vi "Integrated File.vi"() -> ()   [LabVIEW 2021]
uses:
  <vilib>/MakerHub/LINX/Public/Sensors/Accelerometer/MPU60X0/DeviceAddresses.ctl
  <vilib>/MakerHub/LINX/Public/Sensors/Accelerometer/MPU60X0/Clock Source.ctl
  <vilib>/MakerHub/LINX/Public/Utilities/Open Serial.vi
  <vilib>/MakerHub/LINX/Public/Sensors/Motion/Servo/Servo Open One Channel.vi
  <vilib>/MakerHub/LINX/Public/Sensors/Motion/Servo/Servo Close One Channel.vi
  <vilib>/MakerHub/LINX/LMH-LINX.lvlib
  <vilib>/MakerHub/LINX/Public/Sensors/Accelerometer/MPU60X0/MPU60X0.lvlib
  <vilib>/MakerHub/LINX/Public/Sensors/Motion/Servo/Servo.lvlib
panel:
  in  "Ki X":dbl
  in  "Kd X":dbl
  in  "Kp X":dbl=1.0
  in  "Controller Type X":string(combo)="P"
  out "Acc Angle Y":dbl[](graph)=[nan]
  out "Acc Angle X":dbl[](graph)=[131.31801279400403]
  in  "Ki Y":dbl
  in  "Kd Y":dbl
  in  "Kp Y":dbl=1.0
  in  "Controller Type Y":string(combo)="P"
  out "Weighted Angle Y":dbl[](graph)=[nan]
  out "Weighted Angle X":dbl[](graph)=[131.31801279400403]
  in  "Alpha Y":dbl
  in  "Alpha X":dbl
  in  "Acc Offset Y":dbl[](array[numeric])=[90.0]
  in  "Acc Offset X":dbl[](array[numeric])=[30.0]
  in  "Reset":bool
  out "Gyro Angle X":dbl(graph)=10.372999999999987
  out "Gyro Angle Y":dbl(graph)=2.7879999999999896
  in  "Stop Button":bool
  out "Milliseconds to wait out":u32=1
  in  "Milliseconds to wait in":u32=1
  in  "Gyro Offset X":i16
  in  "Gyro Offset Y":i16
  in  "Serial Port":refnum<visa-resource-name>="COM8"
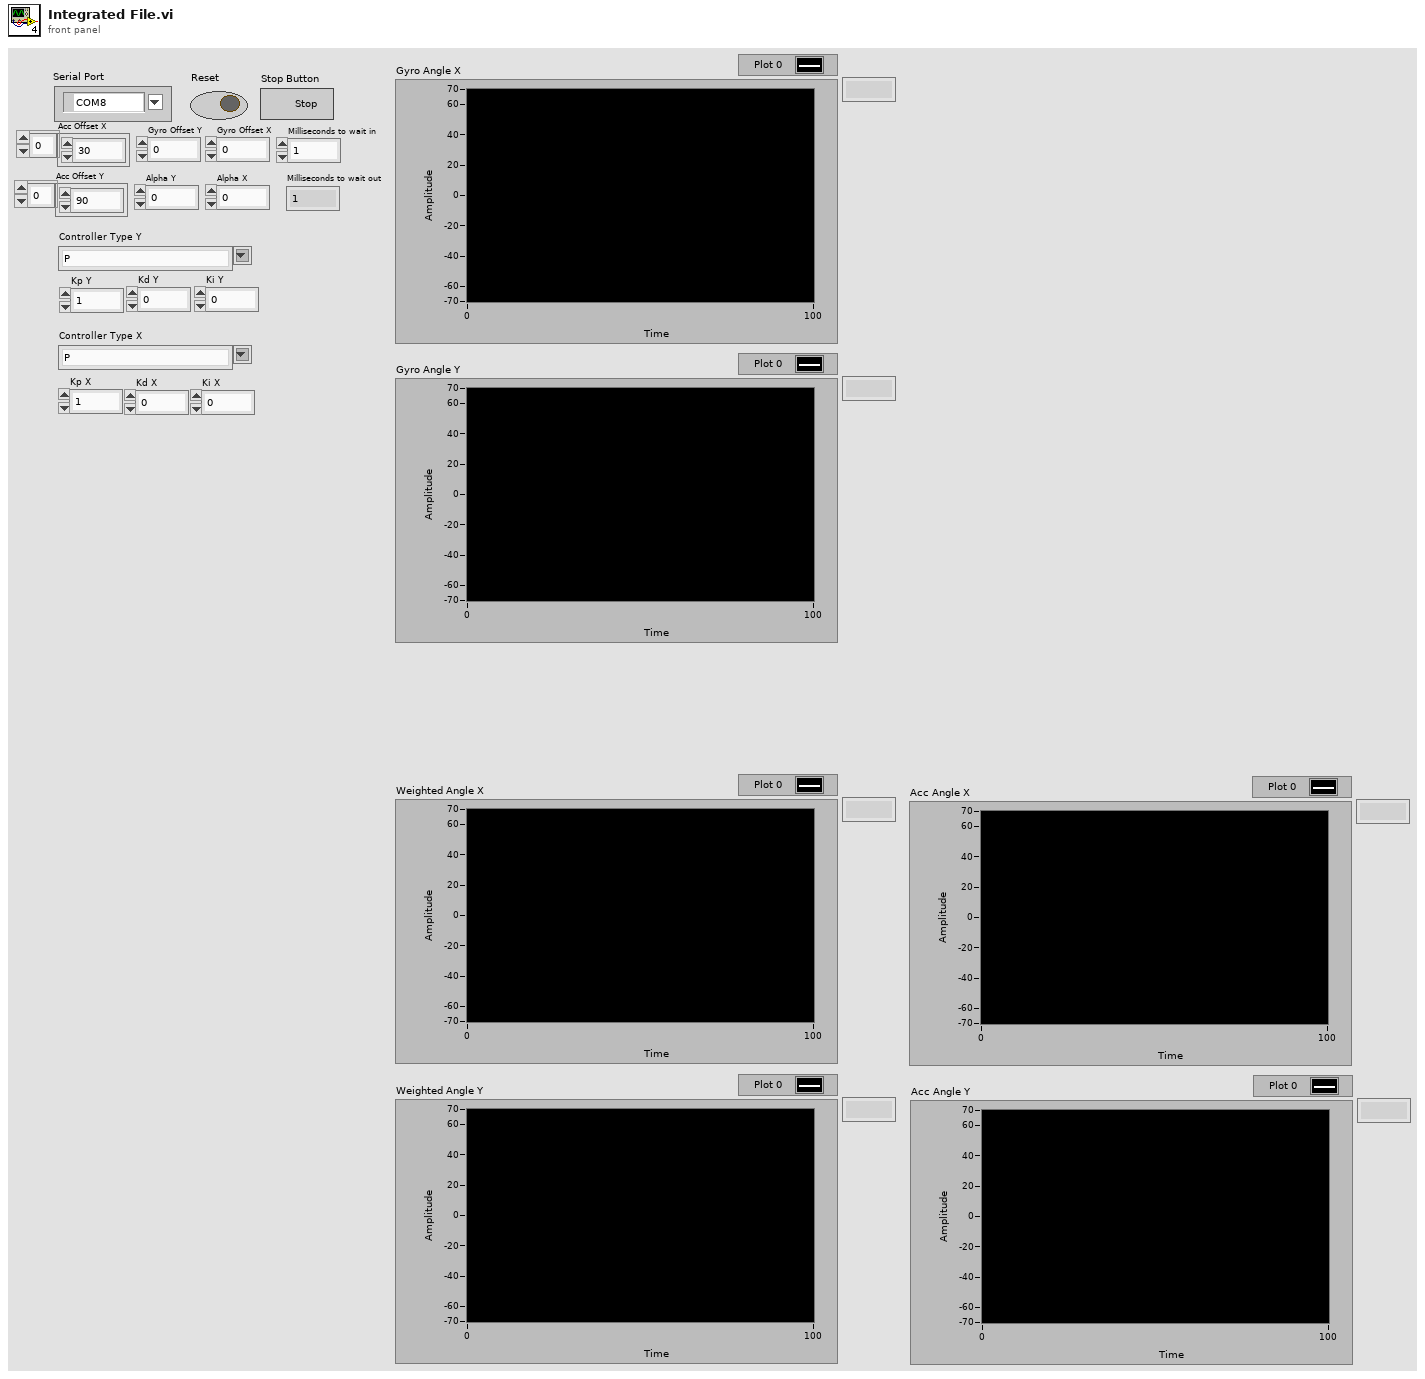
[diagram p1: front panel]
types:
  T1 = typedef "LMH-LINX.lvlib/MPU60X0.lvlib/Clock Source.ctl" = enum8{"Internal 8MHz Osc", "PLL with X Gyro Ref", "PLL with Y Gyro Ref", "PLL with Z Gyro Ref", "PLL with ext 32.768 KHz Ref", "PLL with ext 19.2 MHz Ref", "Reserved", "Hold in reset"}
  T2 = typedef "LMH-LINX.lvlib/MPU60X0.lvlib/DeviceAddresses.ctl" = enum16{"0x68", "0x69"}
  T3 = typedef "LMH-LINX.lvlib/LINX Ref.ctl" = cluster{"IO":T4, "Interface":T5, "LINX Device Config":T6}
  T4 = typedef "LMH-LINX.lvlib/Platform.ctl" = enum16{"Remote", "Local"}
  T5 = typedef "LMH-LINX.lvlib/Interface.ctl" = enum16{"Serial", "TCP"}
  T6 = typedef "LMH-LINX.lvlib/Device.lvlib/LINX Device Config.ctl" = cluster{"Interface":T5, "COM Port":refnum<visa-resource-name>, "TCP Configuration":T7, "Device Family":u8, "Device ID":u8, "Device Name":string, "TCP Ref":refnum<k5>, "Channels":T8}
  T7 = typedef "LMH-LINX.lvlib/Device.lvlib/TCP Config.ctl" = cluster{"IP Address":string, "Port":u16}
  T8 = typedef "LMH-LINX.lvlib/Channels.ctl" = cluster{"DI":u8[], "DO":u8[], "AI":u8[], "AO":u8[], "PWM":u8[], "QE":u8[], "UART":u8[], "I2C 2":u8[], "SPI":u8[], "CAN":u8[], "Servo":u8[], "AI Ref (V)":dbl, "AI Resolution (Bits)":u8, "AO Ref (V)":dbl, "AO Resolution (Bits)":u8}
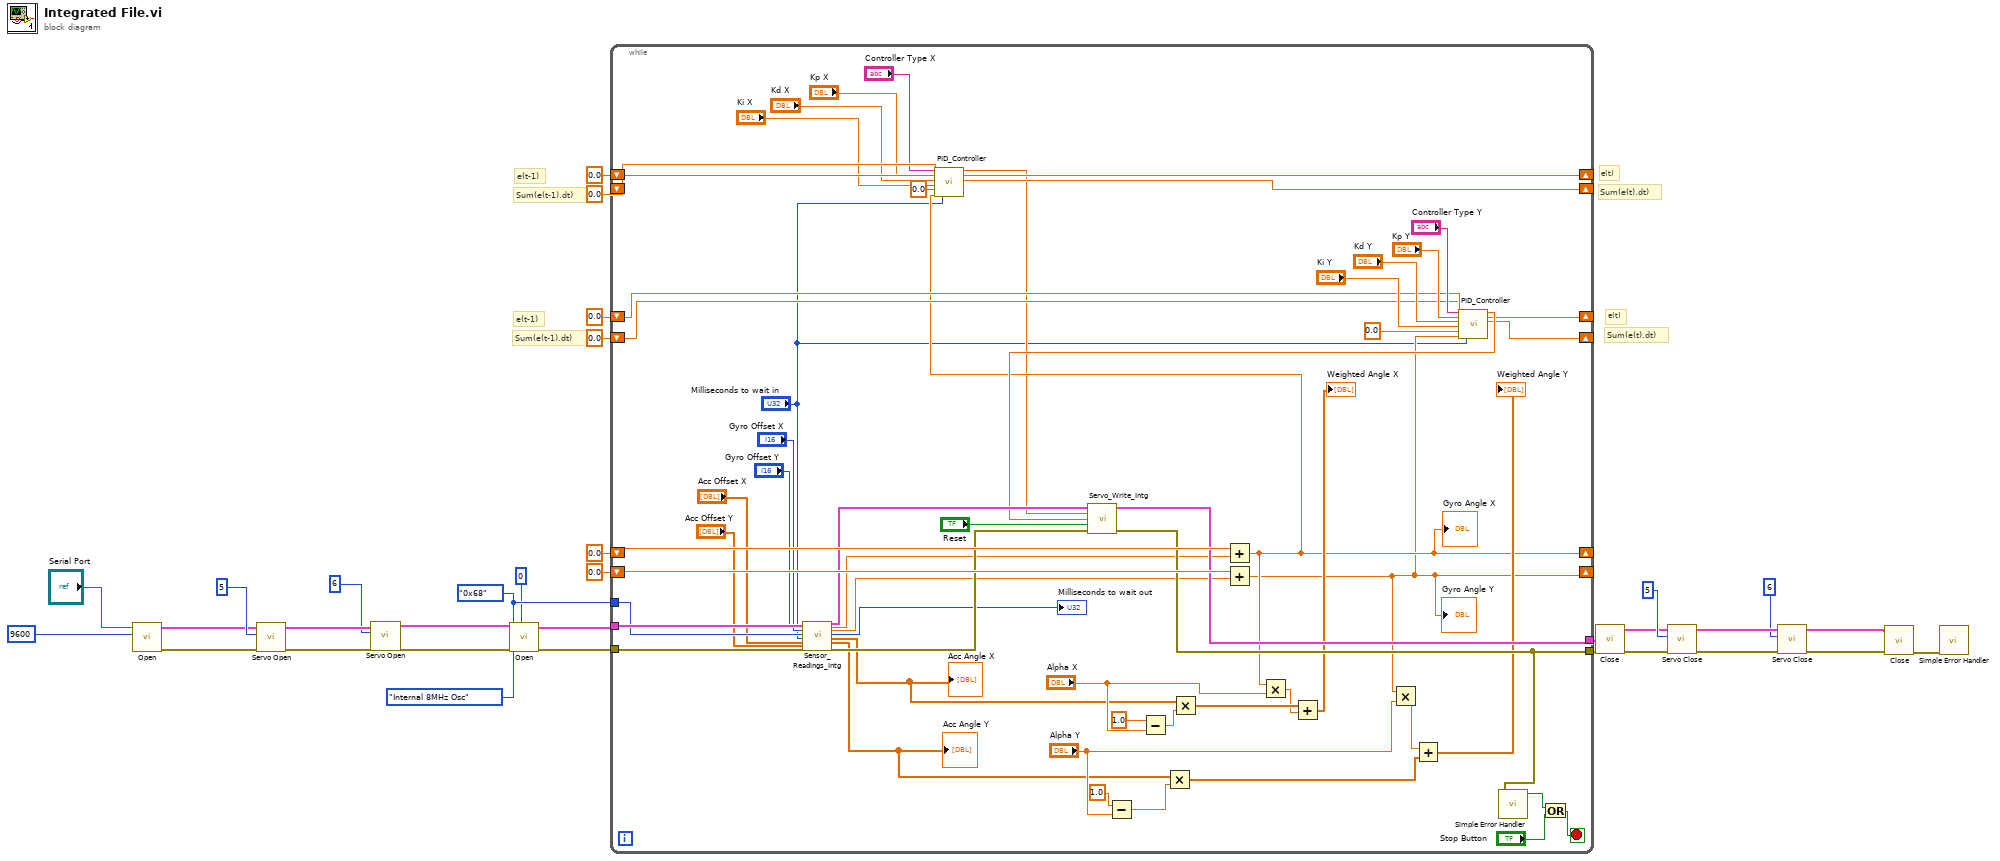
[diagram p0: block diagram]
diagram:
  w27 = DeviceAddresses."0x68" ("I2C Slave Address")
  # "Sum(e(t).dt)"
  # "e(t)"
  # "Sum(e(t-1).dt)"
  # "e(t-1)"
  # "Sum(e(t-1).dt)"
  # "e(t-1)"
  # "Sum(e(t).dt)"
  # "e(t)"
  n1 = call-poly <vilib>:"Open.vi"("Baud Rate Override"=u32 9600, "Serial Port"="Serial Port") -> ("Error Out"=w15:errorcluster, "LINX Resource"=w16:T3)  [unwired: 7 in, 1 out]
  n2 = call-poly <vilib>:"Servo Open.vi"("Error In"=w15, "Servo Channel"=u8 5, "LINX Resource"=w16) -> ("Error Out"=w19:errorcluster, "LINX Resource"=w20:T3)  [unwired: 7 in]
  n3 = call-poly <vilib>:"Servo Open.vi"("Error In"=w19, "Servo Channel"=u8 6, "LINX Resource"=w20) -> ("Error Out"=w13:errorcluster, "LINX Resource"=w14:T3)  [unwired: 7 in]
  n4 = call <vilib>:"Open.vi"("I2C Channel"=u8 0, "Error In"=w13, "Clock Source"=Clock_Source."Internal 8MHz Osc", "I2C Slave Address"=w27, "LINX Resource"=w14) -> ("Error Out"=w28:errorcluster, "LINX Resource"=w29:T3)  [unwired: 5 in]
  n5 = while {
    tunnel: w29 -> [w75]
    tunnel: w28 -> [w74]
    tunnel: w27 -> [w73]
    tunnel: [w84] -> w24
    tunnel: [w83] -> w23
    shift-right: [w36] -> _
    shift-left: 0.0 -> [w86]
    shift-right: [w34] -> _
    shift-left: 0.0 -> [w85]
    shift-right: [w42] -> _
    shift-left: 0.0 ("e(t)") -> [w45]
    shift-right: [w43] -> _
    shift-left: 0.0 ("e(t-1).dt+e(t).dt") -> [w44]
    shift-right: [w49] -> _
    shift-left: 0.0 ("e(t)") -> [w47]
    shift-right: [w48] -> _
    shift-left: 0.0 ("e(t-1).dt+e(t).dt") -> [w46]
    stop <- w87 stop-if-true
    n6 = call "Sensor_Readings_Intg.vi"("LINX Resource in"=w75, "Gyro Offset Y"="Gyro Offset Y", "Gyro Offset X"="Gyro Offset X", "I2C Slave Address"=w73, "Milliseconds to wait in"="Milliseconds to wait in", "Acc Offset X"="Acc Offset X", "Acc Offset Y"="Acc Offset Y", "error in (no error)"=w74) -> ("LINX Resource out"=w68:T3, "Gyro Angle X"=w66:dbl, "Gyro Angle Y"=w65:dbl, "Milliseconds to wait out"=→"Milliseconds to wait out":u32, "Acc Angle X"=w54:dbl[], "Acc Angle Y"=w53:dbl[], "error out"=w67:errorcluster)  [unwired: 13 in]
    "Acc Angle X" <- w54
    "Acc Angle Y" <- w53
    n7 = Subtract(x=1.0, y="Alpha Y") -> (x-y=w77:dbl)
    n8 = Subtract(x=1.0, y="Alpha X") -> (x-y=w81:dbl)
    n9 = Multiply(x=w53, y=w77) -> (x*y=w76:dbl[])
    n10 = Multiply(x=w54, y=w81) -> (x*y=w80:dbl[])
    n11 = Add(x=w86, y=w66) -> (x+y=w36:dbl)
    "Gyro Angle X" <- w36
    n12 = call "PID_Controller.vi"("Controller Type"="Controller Type X", "Kp"="Kp X", "Kd"="Kd X", "Ki"="Ki X", "Setpoint"=0.0, "Feedback Signal"=w36, "e(t-1).dt"=w44, "t"="Milliseconds to wait in", "e(t-1)"=w45) -> ("Control Signal"=w35:dbl, "e(t)"=w42:dbl, "e(t-1).dt+e(t).dt"=w43:dbl)  [unwired: 8 in]
    n13 = Add(x=w85, y=w65) -> (x+y=w34:dbl)
    "Gyro Angle Y" <- w34
    n14 = Multiply(x=w36, y="Alpha X") -> (x*y=w79:dbl)
    n15 = Add(x=w80, y=w79) -> (x+y=→"Weighted Angle X":dbl[])
    n16 = Multiply(x=w34, y="Alpha Y") -> (x*y=w78:dbl)
    n17 = Add(x=w78, y=w76) -> (x+y=→"Weighted Angle Y":dbl[])
    n18 = call "PID_Controller.vi"("Controller Type"="Controller Type Y", "Kp"="Kp Y", "Kd"="Kd Y", "Ki"="Ki Y", "Setpoint"=0.0, "Feedback Signal"=w34, "e(t-1).dt"=w46, "t"="Milliseconds to wait in", "e(t-1)"=w47) -> ("Control Signal"=w56:dbl, "e(t)"=w49:dbl, "e(t-1).dt+e(t).dt"=w48:dbl)  [unwired: 8 in]
    n19 = call "Servo_Write_Intg.vi"("LINX Resource in"=w68, "Servo X"=w35, "Servo Y"=w56, "Reset"="Reset", "error in (no error)"=w67) -> ("LINX Resource out"=w84:T3, "error out"=w83:errorcluster)  [unwired: 9 in]
    n20 = call <vilib>:"Simple Error Handler.vi"("error in (no error)"=w83) -> ("error?"=w89:bool)  [unwired: 4 in, 4 out]
    n21 = Or(x=w89, y="Stop Button") -> (x .or. y?=w87:bool)
  }
  n22 = call <vilib>:"Close.vi"("Error In"=w23, "LINX Resource"=w24) -> ("Error Out"=w7:errorcluster, "LINX Resource"=w8:T3)  [unwired: 8 in]
  n23 = call-poly <vilib>:"Servo Close.vi"("Error In"=w7, "Servo Channel"=u8 5, "LINX Resource"=w8) -> ("Error Out"=w11:errorcluster, "LINX Resource"=w12:T3)  [unwired: 7 in]
  n24 = call-poly <vilib>:"Servo Close.vi"("Error In"=w11, "Servo Channel"=u8 6, "LINX Resource"=w12) -> ("Error Out"=w5:errorcluster, "LINX Resource"=w6:T3)  [unwired: 7 in]
  n25 = call <vilib>:"Close.vi"("Error In"=w5, "LINX Resource"=w6) -> ("Error Out"=w25:errorcluster)  [unwired: 9 in]
  n26 = call <vilib>:"Simple Error Handler.vi"("error in (no error)"=w25) -> ()  [unwired: 4 in, 5 out]
